vi "PDash - Create New DQMH Event.vi"(9 "Ephemeral Scripting Info":T1, 10 "Event Info":T2 {"timeout (ms)" min=-1 step=1}, 11 "Module Info":T5) -> (0 "error out":errorcluster)   [LabVIEW 2019]
doc: "_____\nCreated using DQMH Event Scripter 7.1.0.1447."
uses:
  <vilib>/Delacor/Delacor QMH/Libraries/_Scripting Support/Module Info--cluster.ctl
  <vilib>/Delacor/Delacor QMH/Libraries/_Scripting Support/Module Type--enum.ctl
  <vilib>/Delacor/Delacor QMH/Libraries/_Scripting Support/Event Info (New)--cluster.ctl
  <vilib>/Delacor/Delacor QMH/Libraries/_Scripting Support/Event Type (New)--enum.ctl
  <vilib>/Delacor/Delacor QMH/Libraries/_Scripting Support/Request Scoping--enum.ctl
  <vilib>/Delacor/Delacor QMH/Libraries/_Scripting Support/Ephemeral Scripting Info--cluster.ctl
  PantherDashboard Scripting Hooks/Panther Dasboard Scripting Hooks.lvlib
  <vilib>/Delacor/Delacor QMH/Libraries/_Scripting Support/dqmh_lib_DQMH Scripting Support.lvlib
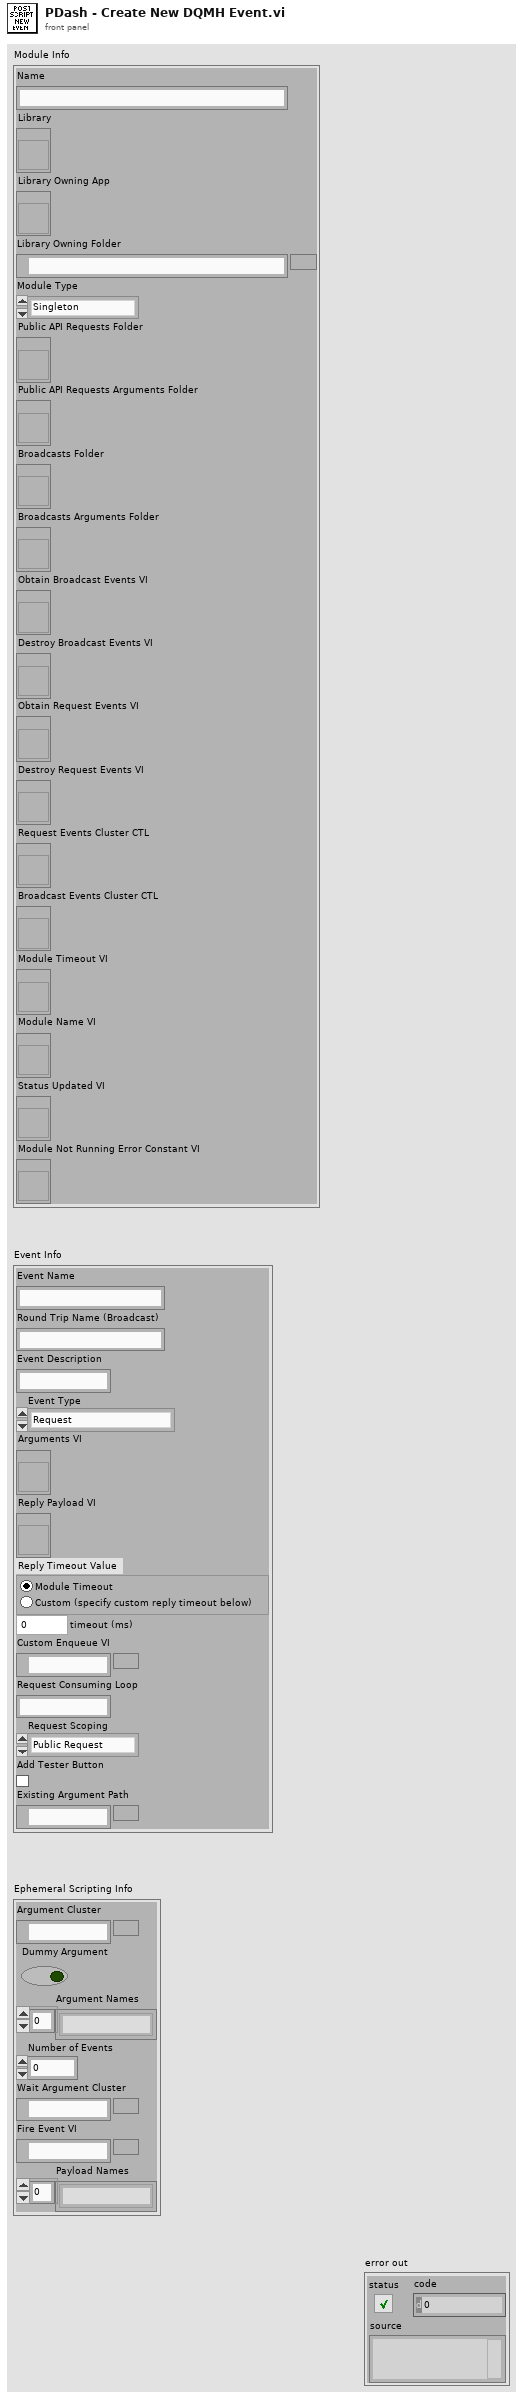
[diagram p1: front panel]
types:
  T1 = typedef "dqmh_lib_DQMH Scripting Support.lvlib/Ephemeral Scripting Info--cluster.ctl" = cluster{"Argument Cluster":path, "Dummy Argument":bool, "Argument Names":string[], "Number of Events":i32, "Wait Argument Cluster":path, "Fire Event VI":path, "Payload Names":string[]}
  T2 = typedef "dqmh_lib_DQMH Scripting Support.lvlib/Event Info (New)--cluster.ctl" = cluster{"Event Name":string, "Round Trip Name (Broadcast)":string, "Event Description":string, "Event Type":T3, "Arguments VI":refnum<vi>, "Reply Payload VI":refnum<vi>, "Reply Timeout Value":enum32{"Module Timeout", "Custom"}, "timeout (ms)":i32, "Custom Enqueue VI":path, "Request Consuming Loop":string, "Request Scoping":T4, "Add Tester Button":bool, "Existing Argument Path":path}
  T3 = typedef "dqmh_lib_DQMH Scripting Support.lvlib/Event Type (New)--enum.ctl" = enum16{"Request", "Broadcast", "Request and Wait for Reply", "Round Trip"}
  T4 = typedef "dqmh_lib_DQMH Scripting Support.lvlib/Request Scoping--enum.ctl" = enum16{"Public Request", "Private Request", "Local Instance"}
  T5 = typedef "dqmh_lib_DQMH Scripting Support.lvlib/Module Info--cluster.ctl" = cluster{"Name":string, "Library":refnum<vi>, "Library Owning App":refnum<vi>, "Library Owning Folder":path, "Module Type":T6, "Public API Requests Folder":refnum<vi>, "Public API Requests Arguments Folder":refnum<vi>, "Broadcasts Folder":refnum<vi>, "Broadcasts Arguments Folder":refnum<vi>, "Obtain Broadcast Events VI":refnum<vi>, "Destroy Broadcast Events VI":refnum<vi>, "Obtain Request Events VI":refnum<vi>, "Destroy Request Events VI":refnum<vi>, "Request Events Cluster CTL":refnum<vi>, "Broadcast Events Cluster CTL":refnum<vi>, "Module Timeout VI":refnum<vi>, "Module Name VI":refnum<vi>, "Status Updated VI":refnum<vi>, "Module Not Running Error Constant VI":refnum<vi>}
  T6 = typedef "dqmh_lib_DQMH Scripting Support.lvlib/Module Type--enum.ctl" = enum16{"Singleton", "Cloneable"}
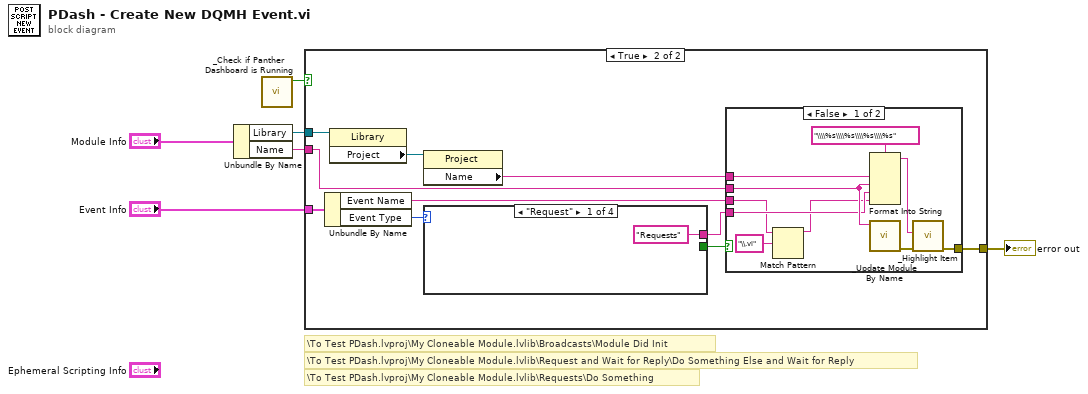
[diagram p0: block diagram]
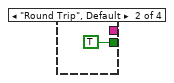
[diagram p4: hidden frame]
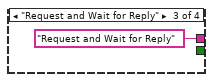
[diagram p5: hidden frame]
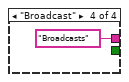
[diagram p6: hidden frame]
diagram:
  # "\\To Test PDash.lvproj\\My Cloneable Module.lvlib\\Requests\\Do Something"
  # "\\To Test PDash.lvproj\\My Cloneable Module.lvlib\\Request and Wait for Reply\\Do Something Else and Wait for Reply"
  # "\\To Test PDash.lvproj\\My Cloneable Module.lvlib\\Broadcasts\\Module Did Init"
  n1 = Unbundle By Name("Module Info") -> ("Library"=w1:refnum<vi>, "Name"=w4:string)
  n2 = call "_Check if Panther Dashboard is Running.vi"() -> ("Panther Dashboard is Running?"=w3:bool)  [unwired: 10 in, 1 out]
  n3 = case shown="True" w3 {
    tunnel: w4 -> [_ w10]
    tunnel: [_ w16] -> w6
    tunnel: "Event Info" -> [_ w15]
    tunnel: w1 -> [_ w14]
    frame False {
    }
    frame True {
      n4 = Unbundle By Name(w15) -> ("Event Name"=w8:string, "Event Type"=w11:T3)
      n5 = property class="Library"(reference=w14) -> ("Project"=w13:refnum<vi>)  [unwired: 1 in, 2 out]
      n6 = property class="Project"(reference=w13) -> ("Name"=w12:string)  [unwired: 1 in, 2 out]
      n7 = case shown="\"Request\"" w11 {
        tunnel: ["Requests" _ "Request and Wait for Reply" "Broadcasts"] -> w9
        tunnel: [_ TRUE _ _] -> w7
        frame "Request" {
        }
        frame "Round Trip", Default {
        }
        frame "Request and Wait for Reply" {
        }
        frame "Broadcast" {
        }
      }
      n8 = case shown="False" w7 {
        tunnel: [w25 _] -> w16
        tunnel: w12 -> [w24 _]
        tunnel: w10 -> [w21 _]
        tunnel: w9 -> [w20 _]
        tunnel: w8 -> [w19 _]
        frame False {
          n9 = Match Pattern(string=w19, regular expression="\\.vi") -> (before substring=w18:string)  [unwired: 1 in, 3 out]
          n10 = Format Into String(format string="\\\\%s\\\\%s\\\\%s\\\\%s", w24, w21, w20, w18) -> (resulting string=w23:string)  [unwired: 2 in, 1 out]
          n11 = call "_Update Module By Name.vi"("Module Name"=w21) -> ("error out"=w26:errorcluster)  [unwired: 10 in]
          n12 = call "_Highlight Item.vi"("error in"=w26, "Item Tag"=w23) -> ("error out"=w25:errorcluster)  [unwired: 9 in]
        }
        frame True {
        }
      }
    }
  }
  "error out" <- w6
